vi "ASE Experiment Control.vi"() -> ()   [LabVIEW 2013]
doc: "This example demonstrates a simple analog loopback."
uses:
  <vilib>/Simulation/Scripting/Companion Diagram/SimConfigNode/SimParams.ctl
  <vilib>/Simulation/Scripting/Companion Diagram/SimConfigNode/_simSolvers.ctl
  <vilib>/Simulation/Implementation/Shared/SIMSCR Execution Mode.ctl
  <vilib>/Simulation/Param Hierarchy/Typedefs/SIMPH Param Control Actions.ctl
  <vilib>/Platform/TimedLoop/XDataNode/timing_clust.ctl
  <vilib>/Platform/TimedLoop/XDataNode/nitl_modes.ctl
  <vilib>/Platform/TimedLoop/XDataNode/wakeup.ctl
  <vilib>/Simulation/Implementation/Shared/SIM limit type.ctl
  <vilib>/Simulation/Implementation/Shared/NILVSim_ParamChanged.vi
  <vilib>/Simulation/Implementation/Shared/NILVSIM_BeginStep.vi
  <vilib>/Simulation/Implementation/Shared/NILVSim_Manager.vi
  <vilib>/Simulation/Implementation/Shared/NILVSim_FinalizeModel.vi
  <vilib>/Simulation/Implementation/Shared/NILVSim_FinishedLate.vi
  <vilib>/Simulation/Utility/Implementation/SIM Halt.vi
  <vilib>/Simulation/SignalArithmetic/Implementation/NILVSim Gain.llb/SIM Gain (scalar).vi
  <vilib>/Simulation/DataSources/Implementation/NILVSim Signal Generator.llb/SIM Signal Generator (scalar).vi
  <vilib>/Simulation/Nonlinear/Implementation/NILVSim Saturation.llb/SIM Saturation (scalar).vi
  <vilib>/Simulation/SignalArithmetic/Implementation/NILVSim Gain.llb/SIM Gain (vector).vi
  <vilib>/Simulation/ContinuousLinear/Implementation/NILVSim Transfer Function.llb/SIM Transfer Function Distributor (MIMO).vi
  <vilib>/Simulation/ContinuousLinear/Implementation/NILVSim Transfer Function.llb/SIM Transfer Function Collector (MIMO).vi
  <vilib>/Simulation/ContinuousLinear/Implementation/NILVSim Transfer Function.llb/SIM Transfer Function Distributor (SISO).vi
  <vilib>/Simulation/ContinuousLinear/Implementation/NILVSim Transfer Function.llb/SIM Transfer Function Collector (SISO).vi
  <vilib>/Simulation/SignalArithmetic/Implementation/NILVSim Gain.llb/SIM Gain (vector,MatrixGain).vi
  <vilib>/Simulation/Nonlinear/Implementation/NILVSim RateLimiter.llb/SIM RateLimiter (scalar).vi
  <vilib>/Simulation/ContinuousLinear/Implementation/NILVSim Integrator new.llb/SIM Integrator distributor (scalar).vi
  <vilib>/Simulation/ContinuousLinear/Implementation/NILVSim Integrator new.llb/SIM Integrator collector (scalar).vi
  <vilib>/Simulation/Nonlinear/Implementation/NILVSim Saturation.llb/SIM Saturation (vector).vi
  <vilib>/Simulation/Implementation/Shared/SIM Unbundle Sim Info.vi
  <vilib>/Utility/error.llb/Clear Errors.vi
  <vilib>/Simulation/Implementation/Shared/NILVSim_GetModelError.vi
  <vilib>/Simulation/Implementation/Shared/SIM Bundle Sim Info.vi
  <vilib>/Simulation/Implementation/Shared/NILVSim_Initialize.vi
  <vilib>/Simulation/Utility/Implementation/NILVSim Get Time and IsAcceptedStep.vi
  <vilib>/Simulation/Implementation/Shared/SIMSH Read Queue.vi
  <vilib>/Simulation/Scripting/Companion Diagram/SimConfigNode/SimDog.xnode
  <vilib>/Simulation/Implementation/XNodeFramework/SimXNode/SimX.xnode
  <vilib>/Quanser/Rapid Control Prototyping Toolkit/hardware/HIL Board/HIL Board.lvclass
  <vilib>/Quanser/Rapid Control Prototyping Toolkit/hardware/HIL Immediate IO/_TypeSpecific/CL HIL Read Analog (Scalar).vi
  <vilib>/Quanser/Rapid Control Prototyping Toolkit/hardware/HIL Immediate IO/CL HIL Read.vi
  <vilib>/Quanser/Rapid Control Prototyping Toolkit/hardware/HIL Immediate IO/CL HIL Read Mixed.vi
  <vilib>/Quanser/Rapid Control Prototyping Toolkit/hardware/HIL Immediate IO/CL HIL Write Mixed.vi
  <vilib>/Quanser/Rapid Control Prototyping Toolkit/hardware/HIL Immediate IO/CL HIL Write.vi
  <vilib>/Platform/TimedLoop/XDataNode/XDataNode.xnode
  <vilib>/Simulation/ContinuousLinear/Implementation/NILVSim Transfer Function.llb/SIM Transfer Function (SISO).vi
  <vilib>/Simulation/ContinuousLinear/Implementation/NILVSim Transfer Function.llb/SIM Transfer Function (MIMO).vi
  <vilib>/Simulation/ContinuousLinear/Implementation/NILVSim Integrator new.llb/SIM Integrator (scalar).vi
  <vilib>/Simulation/Implementation/Shared/NI_SIM_Implementation.lvlib
  <vilib>/Platform/TimedLoop/XDataNode/XDNodeRunTimeDep.lvlib
panel:
  in  "k4":dbl(slide) scale=-100.0..100.0
  in  "k3":dbl(slide) scale=-100.0..100.0
  in  "k2":dbl(slide)=29.55974842767295 scale=-100.0..100.0
  in  "k1":dbl(slide)=1.886792452830184 scale=-100.0..100.0
  in  "Setpoint Command":T1={"Amplitude (m)"=0.01, "Frequency (Hz)"=0.3} caption="Road (Bottom Plate)\nAmplitude Command (m)" {"Frequency (Hz)" min=0.0 max=0.5 step=0.009999999776482582 format="%_3f"; "Amplitude (m)" min=-10.0 max=10.0 step=0.5 format="%_3f"}
  out "Active Suspension Motor Voltage (V)":dbl(graph)
  out "?":string="Active Suspension (Closed Loop)"
  in  "Control Mode":bool
  out "Zr(m), Zs(m), Zus(m)":T2(graph)={"output"=0.0096065956, "Result"=0.0090666584, "output"=0.0091514816}
  out "Accelerometer Signal":dbl[](graph)=[0.003882702641658684]
  in  "Halt?":bool
  # "Active Suspension Experiment"
  # "Select the data acquisition card in the HIL Initialize VI on the block diagram.\n\nFollow connections given in Lab Manual.\n\nRun this VI.\n\nZr represents the bottom plate position which refers to the road. Zus represents the middle plate position which refers to vehicle tire. Zs represents the top plate position which refers to vehicle body. The bias voltage due to gravity is removed from the accelerometer measurement. \n\nManually tune the control gains based on the simulation results. You can either use the sliders or type in the gain values. A sample set of gains are set by default.\n\nSwitch between the open loop (passive suspension) and closed loop (active suspension) control using the Control Mode button.\n\nStop the VI by pressing the Stop button.\n\nDisclaimer: Due to inherent friction and nonlinear effects in the system the signals that are measured and monitored by the user might slightly vary from the ones shown in the documentation."
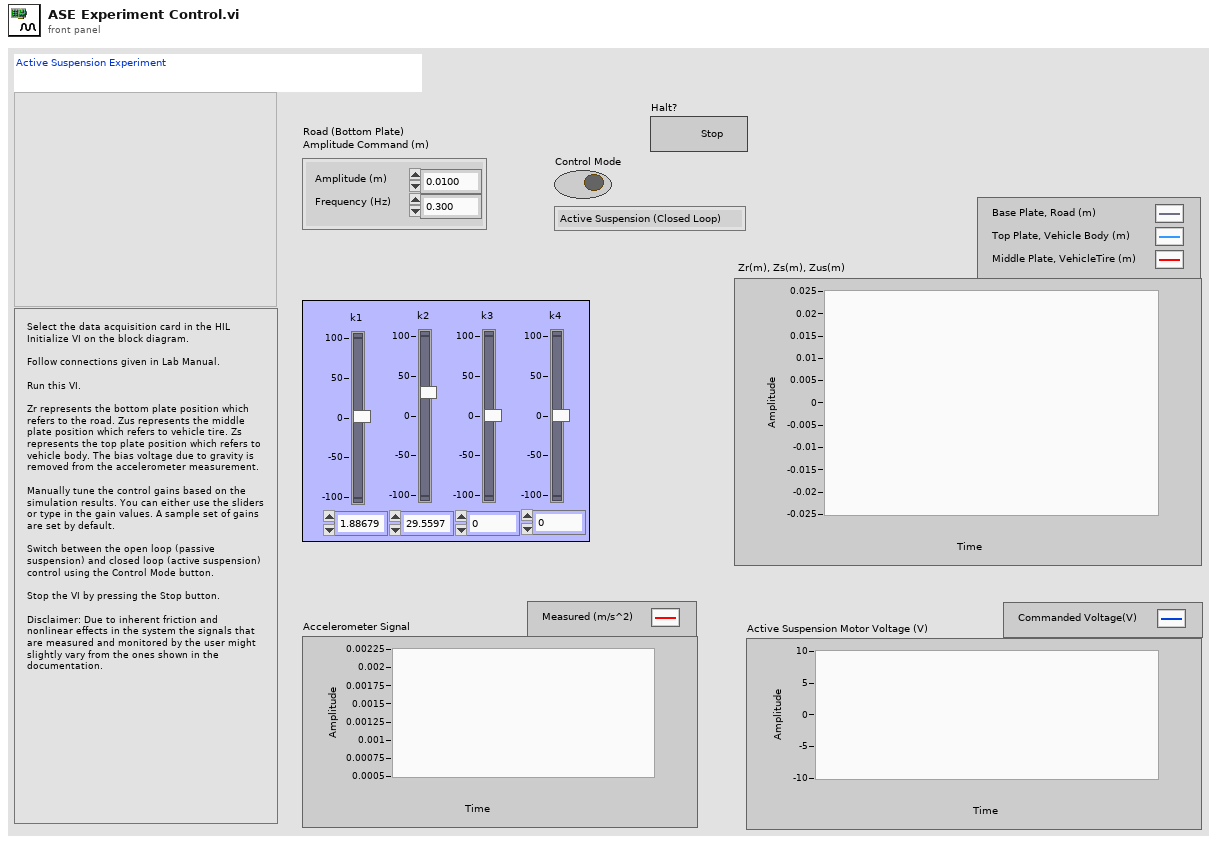
[diagram p1: front panel]
types:
  T1 = cluster{"Amplitude (m)":dbl, "Frequency (Hz)":dbl}
  T2 = cluster{"output":dbl, "Result":dbl, "output":dbl}
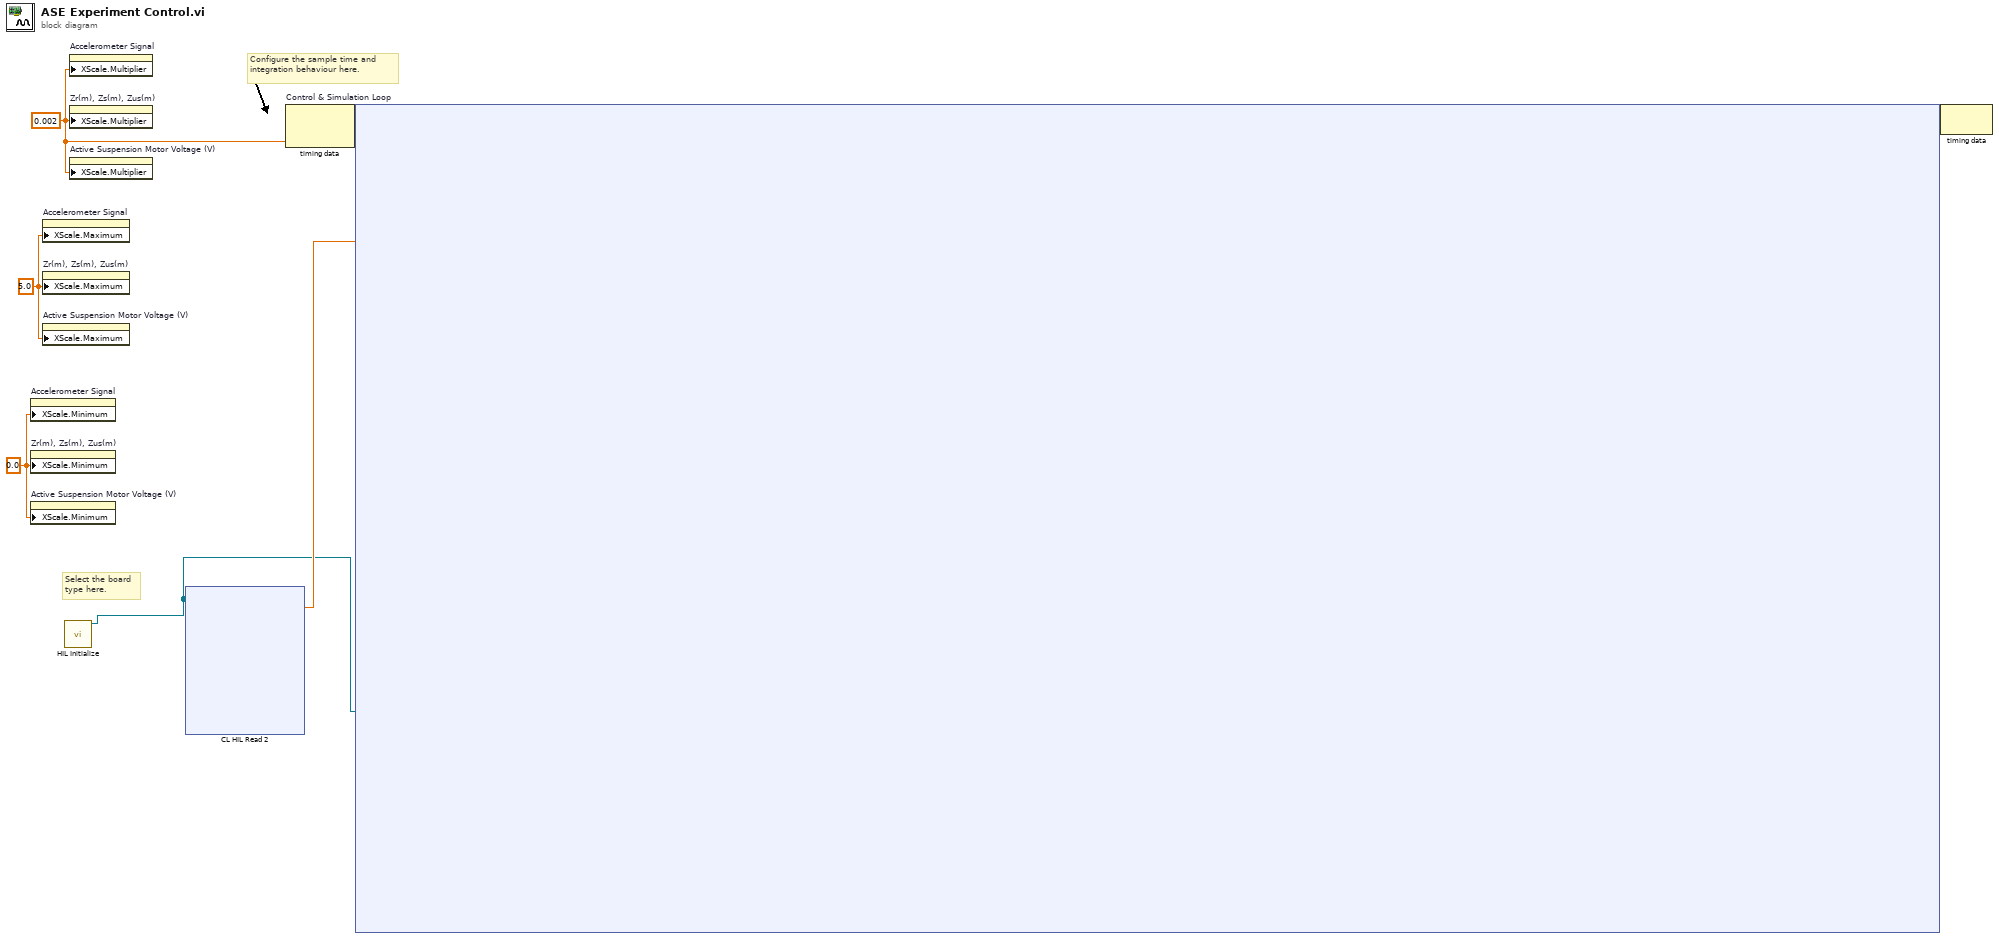
[diagram p0: block diagram]
diagram:
  w1 = 0.002 ("X Scale.Offset and Multiplier:Multiplier")
  w3 = 0.0 ("X Scale.Range:Minimum")
  w4 = 5.0 ("X Scale.Range:Maximum")
  # "Configure the sample time and integration behaviour here."
  # "Select the board\ntype here."
  n1 = property on="Accelerometer Signal" class="WFChart (strict)"("XScale.Minimum"=w3) -> ()  [unwired: 2 in, 2 out]
  n2 = property on="Zr(m), Zs(m), Zus(m)" class="WFChart (strict)"("XScale.Minimum"=w3) -> ()  [unwired: 2 in, 2 out]
  n3 = property on="Active Suspension Motor Voltage (V)" class="WFChart (strict)"("XScale.Minimum"=w3) -> ()  [unwired: 2 in, 2 out]
  n4 = property on="Accelerometer Signal" class="WFChart (strict)"("XScale.Maximum"=w4) -> ()  [unwired: 2 in, 2 out]
  n5 = property on="Zr(m), Zs(m), Zus(m)" class="WFChart (strict)"("XScale.Maximum"=w4) -> ()  [unwired: 2 in, 2 out]
  n6 = property on="Active Suspension Motor Voltage (V)" class="WFChart (strict)"("XScale.Maximum"=w4) -> ()  [unwired: 2 in, 2 out]
  n7 = call "HIL Initialize"() -> ("board out"=w2:refnum<class "HIL Board.lvclass">)  [unwired: 14 in, 1 out]
  n8 = property on="Accelerometer Signal" class="WFChart (strict)"("XScale.Multiplier"=w1) -> ()  [unwired: 2 in, 2 out]
  n9 = property on="Zr(m), Zs(m), Zus(m)" class="WFChart (strict)"("XScale.Multiplier"=w1) -> ()  [unwired: 2 in, 2 out]
  n10 = property on="Active Suspension Motor Voltage (V)" class="WFChart (strict)"("XScale.Multiplier"=w1) -> ()  [unwired: 2 in, 2 out]
  n11 = xnode "CL HIL Read 2"("board in"=w2) -> ("analog voltage"=w5:dbl)  [unwired: 2 in, 18 out]
  n12 = node-c288(w1) -> (w7:variant)  [unwired: 1 in]
  n13 = node-c254 "Control & Simulation Loop"(w7, w2, w5) -> (w6:variant)
  n14 = node-c288(w6) -> ()  [unwired: 1 out]
